vi "Server Cmd Answer - Get Status.vi"(6 "error message in":errorcluster, 7 "server event ref":refnum<vi>, 8 "error in":errorcluster, 11 "Status ready? (False)":bool) -> (0 "error out":errorcluster, 3 "info data out":string, 4 "error message out":errorcluster)   [LabVIEW 2020]
doc: "Send answer for command \"Get status\". Optionally clears input error."
uses:
  Server Client Request.ctl
  octave/infolib/String.vi
  octave/infolib/1D String.vi
  octave/infolib/GetBoolean.vi
  octave/infolib/infolib.lvlib
panel:
  in  "client request":T1={"info data"="", "answer handle"=-1}
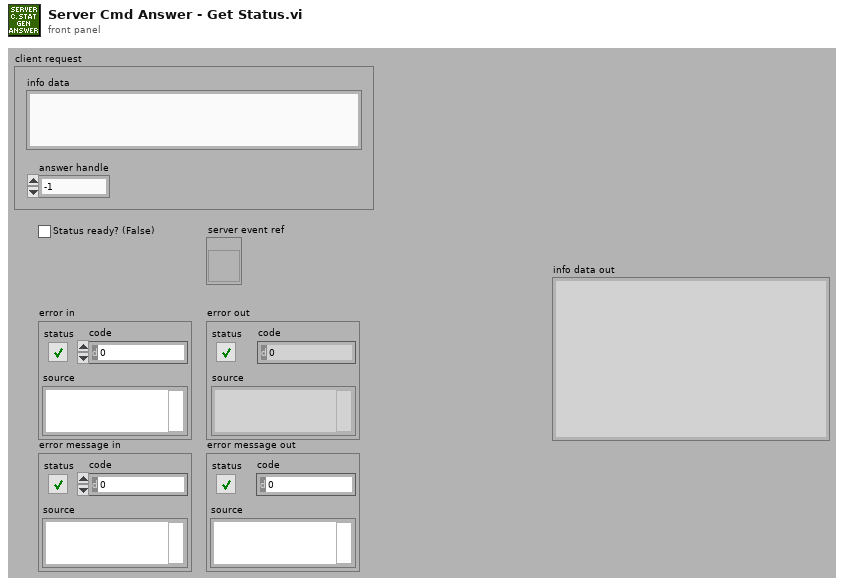
[diagram p1: front panel]
types:
  T1 = typedef "Server Client Request.ctl" = cluster{"info data":string, "answer handle":i32}
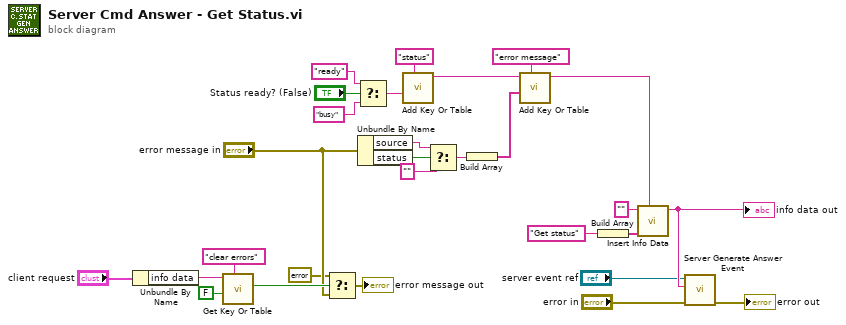
[diagram p0: block diagram]
diagram:
  n1 = Unbundle By Name("client request") -> ("info data"=w6:string)
  n2 = call-poly "Get Key Or Table.vi"("key description"="clear errors", "boolean"=FALSE, "info data"=w6) -> ("value"=w4:bool)  [unwired: 5 in, 3 out]
  n3 = Select(t=errorcluster {"status"=FALSE, "code"=0, "source"=""}, s=w4, f="error message in") -> (s? t:f=→"error message out":errorcluster)
  n4 = Select(t="ready" ("string"), s="Status ready? (False)", f="busy" ("string")) -> (s? t:f=w14:string)
  n5 = Unbundle By Name("error message in") -> ("source"=w12:string, "status"=w13:bool)
  n6 = call-poly "Add Key Or Table.vi"("key description"="status", "string"=w14) -> ("info data out"=w26:string)  [unwired: 8 in, 1 out]
  n7 = Select(t=w12, s=w13, f="") -> (s? t:f=w10:string)
  n8 = Build Array(w10) -> (w9:string[])
  n9 = call-poly "Add Key Or Table.vi"("key description"="error message", "string"=w9, "info data"=w26) -> ("info data out"=w25:string)  [unwired: 7 in, 1 out]
  n10 = Build Array("Get status" ("key description")) -> (w24:string[])
  n11 = call "Insert Info Data.vi"("info data to insert"=w25, "sections"=w24, "info data"="") -> ("info data out"=w22:string)  [unwired: 7 in, 1 out]
  "info data out" <- w22
  n12 = call "Server Generate Answer Event.vi"("error in"="error in", "event data"=w22, "server event ref"="server event ref") -> ("error out"=→"error out":errorcluster)  [unwired: 8 in]
